vi "runtest Find Run for Sparameter.vi"(4 "Save Results?":bool, 5 "Connection Refnum":T1, 6 "Run ID":string, 8 "error in (no error)":errorcluster, 9 "Test ID":string, 10 "Fields":T3[](array[typedef])=[{"ixField"=0, "iSequenceOrder"=0, "sxFieldId"="Serial Number", "sxSequenceId"="", "sDisplayName"="test", "sValue"="", "sUnits"="", "nDataType"=enum."timestamp", "nNextItem"=enum."Reset", "fSystem"=FALSE, "fSystemValue"=FALSE, "fRequired"=FALSE, "fSetAtTest"=FALSE, "fTestField"=FALSE, "fDeleted"=FALSE, "fIndexed"=FALSE, "fFreeList"=FALSE}, {"ixField"=0, "iSequenceOrder"=0, "sxFieldId"="Model Number", "sxSequenceId"="", "sDisplayName"="test", "sValue"="", "sUnits"="", "nDataType"=enum."timestamp", "nNextItem"=enum."Reset", "fSystem"=FALSE, "fSystemValue"=FALSE, "fRequired"=FALSE, "fSetAtTest"=FALSE, "fTestField"=FALSE, "fDeleted"=FALSE, "fIndexed"=FALSE, "fFreeList"=FALSE}], 11 "Data File Path":path) -> (0 "error out":errorcluster, 2 "Current Run":T2, 3 "runs to use":T2[](array[typedef]))   [LabVIEW 2011]
uses:
  _cgi-lib/TDM_INDEX Record.ctl
  server/database/Fields/Field Record.ctl
  server/database/Fields/Field DataTypes.ctl
  server/database/Fields/Field NextItem.ctl
  Summitek EXT/ODBC/SQL Controls/Connection Refnum.ctl
  Summitek EXT/OpenG EXT/file/file.llb/File Exists - Scalar__ogtk.vi
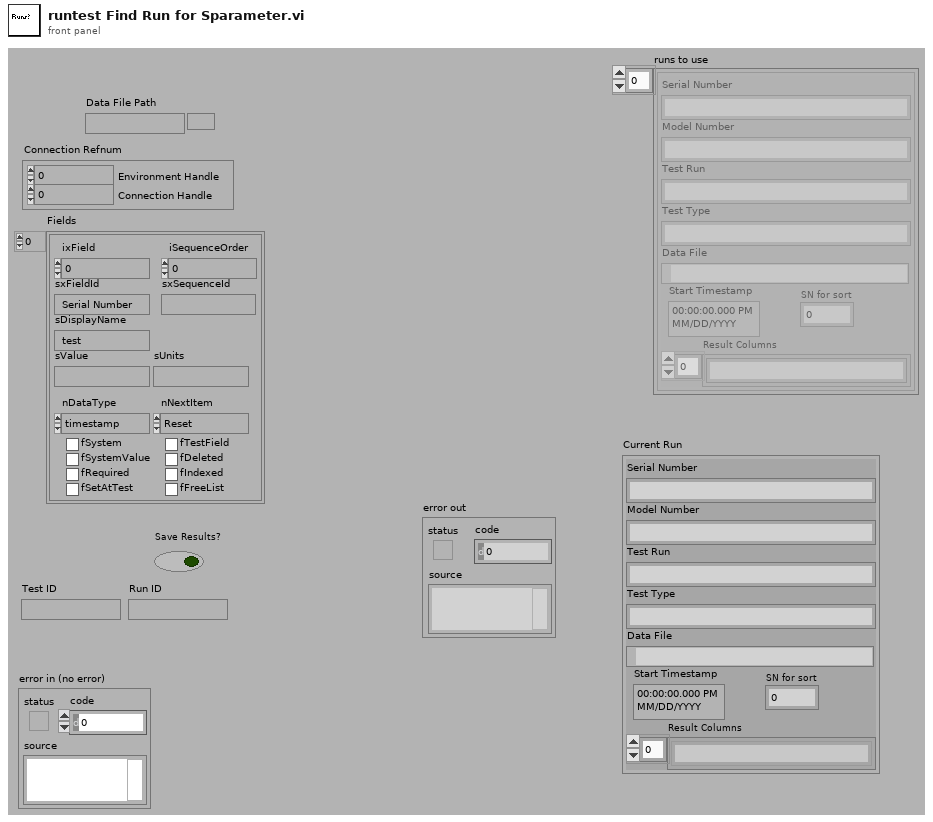
[diagram p1: front panel]
types:
  T1 = typedef "Connection Refnum.ctl" = cluster{"Environment Handle":i32, "Connection Handle":i32}
  T2 = typedef "TDM_INDEX Record.ctl" = cluster{"Model Number":string, "SN for sort":i32, "Test Type":string, "Test Run":string, "Serial Number":string, "Start Timestamp":timestamp, "Data File":path, "Result Columns":string[]}
  T3 = typedef "Field Record.ctl" = cluster{"ixField":i32, "iSequenceOrder":i32, "sxFieldId":string, "sxSequenceId":string, "sDisplayName":string, "sValue":string, "sUnits":string, "nDataType":T4, "nNextItem":T5, "fSystem":bool, "fSystemValue":bool, "fRequired":bool, "fSetAtTest":bool, "fTestField":bool, "fDeleted":bool, "fIndexed":bool, "fFreeList":bool}
  T4 = typedef "Field DataTypes.ctl" = enum32{"text", "numeric", "list", "timestamp", "boolean"}
  T5 = typedef "Field NextItem.ctl" = enum32{"Reset", "Retain", "Auto-Increment"}
  T6 = enum16{"open", "open or create", "create or replace", "create", "open (read-only)"}
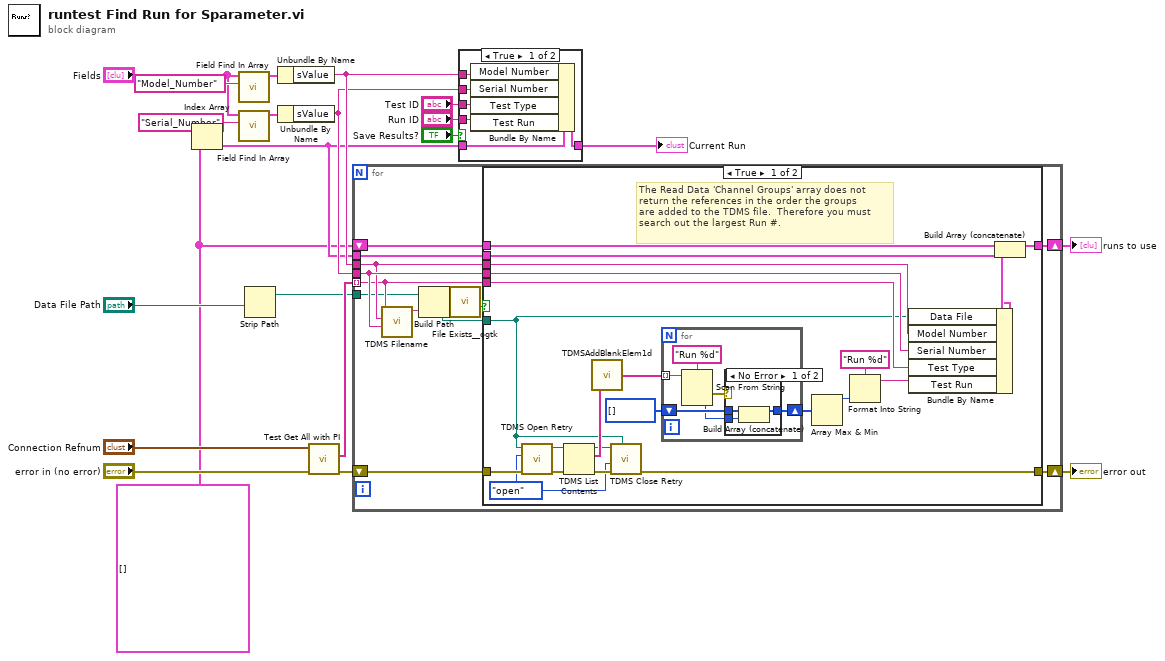
[diagram p0: block diagram]
diagram:
  w1 = T2[] []
  n1 = Index Array(array=w1) -> (element=w2:T2)  [unwired: 1 in]
  n2 = call "Field Find In Array.vi"("FieldID or Display Name(\"\")"="Model_Number" ("Field Internal ID"), "Field Array"="Fields") -> ("Field"=w18:T3)  [unwired: 1 in, 8 out]
  n3 = call "Field Find In Array.vi"("FieldID or Display Name(\"\")"="Serial_Number" ("Field Internal ID"), "Field Array"="Fields") -> ("Field"=w21:T3)  [unwired: 1 in, 8 out]
  n4 = Strip Path(path="Data File Path") -> (stripped path=w3:path)  [unwired: 1 out]
  n5 = Unbundle By Name(w18) -> ("sValue"=w7:string)
  n6 = Unbundle By Name(w21) -> ("sValue"=w6:string)
  n7 = call "Test Get All with PI.vi"("error out"="error in (no error)", "Connection Refnum"="Connection Refnum") -> ("error out 2"=w5:errorcluster, "tests"=w8:string[])  [unwired: 7 in, 1 out]
  n8 = for {
    tunnel: w8 -> [w27] mode=indexing
    tunnel: w7 -> [w28]
    tunnel: w6 -> [w29]
    shift-right: [w33] -> w14
    shift-left: w1 -> [w32]
    shift-right: [w31] -> w15
    shift-left: w5 -> [w23]
    tunnel: w2 -> [w30]
    tunnel: w3 -> [w22]
    n9 = call "TDMS Filename.vi"("Serial Number"=w29, "Model Number"=w28, "Test Type"=w27) -> ("Filename"=w26:string)  [unwired: 8 in]
    n10 = Build Path(base path=w22, name or relative path=w26) -> (appended path=w24:path)
    n11 = call-poly "File Exists__ogtk.vi"("file path"=w24) -> ("exists"=w25:bool)  [unwired: 6 in, 1 out]
    n12 = case shown="True" w25 {
      tunnel: [w45 w67] -> w33
      tunnel: w32 -> [w47 w67]
      tunnel: [w44 w66] -> w31
      tunnel: w23 -> [w55 w66]
      tunnel: w28 -> [w50 _]
      tunnel: w29 -> [w49 _]
      tunnel: w27 -> [w48 _]
      tunnel: w30 -> [w46 _]
      tunnel: w24 -> [w34 _]
      frame True {
        w41 = T6."open" ("operation (0:open)")
        # "The Read Data 'Channel Groups' array does not\nreturn the references in the order the groups\nare added to the TDMS file.  Therefore you must\nsearch out the largest Run #."
        n13 = call "TDMS Open Retry.vi"("error in (no error)"=w55, "Operation (0:open)"=w41, "Path"=w34) -> ("error out"=w54:errorcluster, "TDMS File Ref"=w53:refnum<k34>)  [unwired: 1 in, 6 out]
        n14 = TDMS List Contents(4:w54, 7:w53) -> (0:w42:errorcluster, 2:w52:string[], 3:w43:refnum<k34>)  [unwired: 2 out]
        n15 = call <vilib>:"TDMSAddBlankElem1d.vi"("input string array"=w52) -> ("output string array with blank element at the beginning"=w51:string[])
        n16 = call "TDMS Close Retry.vi"("TDMS Path"=w34, "error in (no error)"=w42, "Operation (0:open)"=w41, "TDMS File Ref"=w43) -> ("error out"=w44:errorcluster)  [unwired: 5 in, 2 out]
        n17 = for {
          tunnel: w51 -> [w60] mode=indexing
          shift-right: [w58] -> w40
          shift-left: i32[] [] -> [w57]
          n18 = Scan From String(format string="Run %d", input string=w60) -> (error out=w59:errorcluster, output 1=w56:i32)  [unwired: 2 in, 3 out]
          n19 = case shown="No Error" w59 {
            tunnel: [w64 w65] -> w58
            tunnel: w57 -> [w63 w65]
            tunnel: w56 -> [w62 _]
            frame No Error {
              n20 = Build Array (concatenate)(w63, w62) -> (w64:i32[])
            }
            frame Error {
            }
          }
        }
        n21 = Array Max & Min(array=w40) -> (max value=w37:i32)  [unwired: 3 out]
        n22 = Format Into String(format string="Run %d", w37) -> (resulting string=w38:string)  [unwired: 2 in, 1 out]
        n23 = Bundle By Name(cluster=w46, "Data File"=w34, "Model Number"=w50, "Serial Number"=w49, "Test Type"=w48, "Test Run"=w38) -> (w36:T2)
        n24 = Build Array (concatenate)(w47, w36) -> (w45:T2[])
      }
      frame False {
      }
    }
  }
  "runs to use" <- w14
  "error out" <- w15
  n25 = case shown="True" "Save Results?" {
    tunnel: w7 -> [w73 _]
    tunnel: w6 -> [w72 _]
    tunnel: "Test ID" -> [w71 _]
    tunnel: "Run ID" -> [w70 _]
    tunnel: w2 -> [w69 w74]
    tunnel: [w68 w74] -> w11
    frame True {
      n26 = Bundle By Name(cluster=w69, "Model Number"=w73, "Serial Number"=w72, "Test Type"=w71, "Test Run"=w70) -> (w68:T2)
    }
    frame False {
    }
  }
  "Current Run" <- w11
